vi "SetUpHelper.vi"(8 "ErrorIn":errorcluster, 9 "EnableCluster":T2, 11 "Reference":T1) -> (0 "ErrorOut":errorcluster, 3 "Reference":T1)   [LabVIEW 2022 SP3]
uses:
  C:/Users/Robots/Documents/robocadSimLV/assemblies/LibraryForLabVIEW.dll
  assemblies/LibraryForLabVIEW.dll
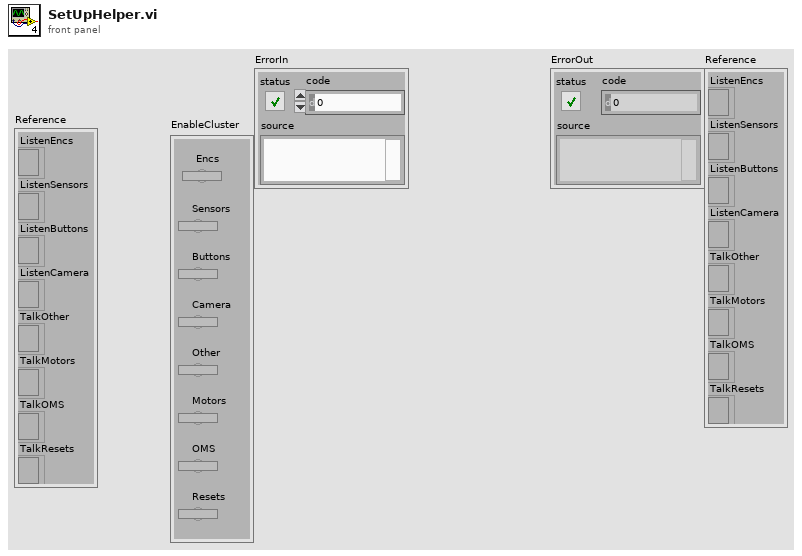
[diagram p1: front panel]
types:
  T1 = cluster{"ListenEncs":refnum<k24>, "ListenSensors":refnum<k24>, "ListenButtons":refnum<k24>, "ListenCamera":refnum<k24>, "TalkOther":refnum<k24>, "TalkMotors":refnum<k24>, "TalkOMS":refnum<k24>, "TalkResets":refnum<k24>}
  T2 = cluster{"Encs":bool, "Sensors":bool, "Buttons":bool, "Camera":bool, "Other":bool, "Motors":bool, "OMS":bool, "Resets":bool}
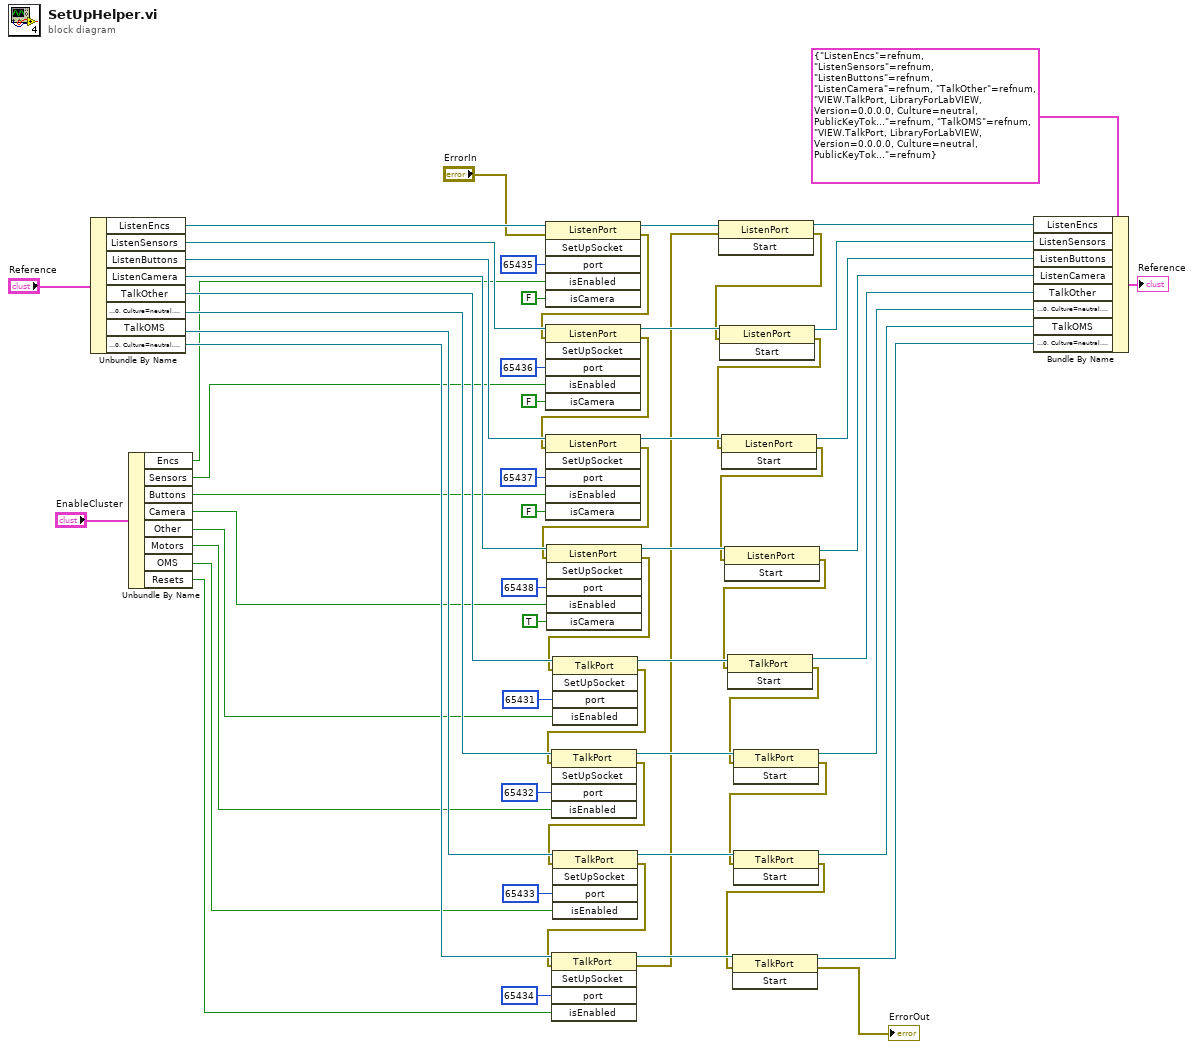
[diagram p0: block diagram]
diagram:
  n1 = Unbundle By Name("Reference") -> ("ListenEncs"=w64:refnum<k24>, "ListenSensors"=w59:refnum<k24>, "ListenButtons"=w56:refnum<k24>, "ListenCamera"=w53:refnum<k24>, "TalkOther"=w50:refnum<k24>, "TalkMotors"=w48:refnum<k24>, "TalkOMS"=w46:refnum<k24>, "TalkResets"=w44:refnum<k24>)
  n2 = Unbundle By Name("EnableCluster") -> ("Encs"=w43:bool, "Sensors"=w42:bool, "Buttons"=w41:bool, "Camera"=w40:bool, "Other"=w39:bool, "Motors"=w38:bool, "OMS"=w37:bool, "Resets"=w36:bool)
  n3 = invoke class="ListenPort" method="SetUpSocket"(reference=w64, error in="ErrorIn", "port"=65435, "isEnabled"=w43, "isCamera"=FALSE) -> (reference out=w27:refnum<k24>, error out=w34:errorcluster)  [unwired: 1 in, 4 out]
  n4 = invoke class="ListenPort" method="SetUpSocket"(reference=w59, error in=w34, "port"=65436, "isEnabled"=w42, "isCamera"=FALSE) -> (reference out=w26:refnum<k24>, error out=w33:errorcluster)  [unwired: 1 in, 4 out]
  n5 = invoke class="ListenPort" method="SetUpSocket"(reference=w56, error in=w33, "port"=65437, "isEnabled"=w41, "isCamera"=FALSE) -> (reference out=w25:refnum<k24>, error out=w32:errorcluster)  [unwired: 1 in, 4 out]
  n6 = invoke class="ListenPort" method="SetUpSocket"(reference=w53, error in=w32, "port"=65438, "isEnabled"=w40, "isCamera"=TRUE) -> (reference out=w24:refnum<k24>, error out=w31:errorcluster)  [unwired: 1 in, 4 out]
  n7 = invoke class="TalkPort" method="SetUpSocket"(reference=w50, error in=w31, "port"=65431, "isEnabled"=w39) -> (reference out=w23:refnum<k24>, error out=w30:errorcluster)  [unwired: 1 in, 3 out]
  n8 = invoke class="TalkPort" method="SetUpSocket"(reference=w48, error in=w30, "port"=65432, "isEnabled"=w38) -> (reference out=w22:refnum<k24>, error out=w29:errorcluster)  [unwired: 1 in, 3 out]
  n9 = invoke class="TalkPort" method="SetUpSocket"(reference=w46, error in=w29, "port"=65433, "isEnabled"=w37) -> (reference out=w21:refnum<k24>, error out=w28:errorcluster)  [unwired: 1 in, 3 out]
  n10 = invoke class="TalkPort" method="SetUpSocket"(reference=w44, error in=w28, "port"=65434, "isEnabled"=w36) -> (reference out=w20:refnum<k24>, error out=w19:errorcluster)  [unwired: 1 in, 3 out]
  n11 = invoke class="ListenPort" method="Start"(reference=w27, error in=w19) -> (reference out=w9:refnum<k24>, error out=w18:errorcluster)  [unwired: 1 in, 1 out]
  n12 = invoke class="ListenPort" method="Start"(reference=w26, error in=w18) -> (reference out=w8:refnum<k24>, error out=w17:errorcluster)  [unwired: 1 in, 1 out]
  n13 = invoke class="ListenPort" method="Start"(reference=w25, error in=w17) -> (reference out=w7:refnum<k24>, error out=w16:errorcluster)  [unwired: 1 in, 1 out]
  n14 = invoke class="ListenPort" method="Start"(reference=w24, error in=w16) -> (reference out=w6:refnum<k24>, error out=w15:errorcluster)  [unwired: 1 in, 1 out]
  n15 = invoke class="TalkPort" method="Start"(reference=w23, error in=w15) -> (reference out=w5:refnum<k24>, error out=w14:errorcluster)  [unwired: 1 in, 1 out]
  n16 = invoke class="TalkPort" method="Start"(reference=w22, error in=w14) -> (reference out=w4:refnum<k24>, error out=w13:errorcluster)  [unwired: 1 in, 1 out]
  n17 = invoke class="TalkPort" method="Start"(reference=w21, error in=w13) -> (reference out=w3:refnum<k24>, error out=w12:errorcluster)  [unwired: 1 in, 1 out]
  n18 = invoke class="TalkPort" method="Start"(reference=w20, error in=w12) -> (reference out=w2:refnum<k24>, error out=→"ErrorOut":errorcluster)  [unwired: 1 in, 1 out]
  n19 = Bundle By Name(cluster=T1 {"ListenEncs"=refnum, "ListenSensors"=refnum, "ListenButtons"=refnum, "ListenCamera"=refnum, "TalkOther"=refnum, "TalkMotors"=refnum, "TalkOMS"=refnum, "TalkResets"=refnum}, "ListenEncs"=w9, "ListenSensors"=w8, "ListenButtons"=w7, "ListenCamera"=w6, "TalkOther"=w5, "TalkMotors"=w4, "TalkOMS"=w3, "TalkResets"=w2) -> (→"Reference":T1)
